vi "662xA Display Text.vi"(8 "error in (no error)":errorcluster, 9 "text message (TEST)":string="TEST", 10 "function (T:write)":bool=TRUE, 11 "VISA resource name":refnum<visa-resource-name>) -> (0 "error out":errorcluster, 3 "VISA resource name out":refnum<visa-resource-name>)   [LabVIEW 2020, in "Agilent 6XXX Series.lvlib"]
doc: "This function displays a text message on the front panel of the HP662XA series power supplies only."
uses:
  <instrlib>/Agilent 6XXX Series/Agilent 6XXX Series.lvlib
panel:
  # "HP662XA series only"
  # "write message\nclear message"
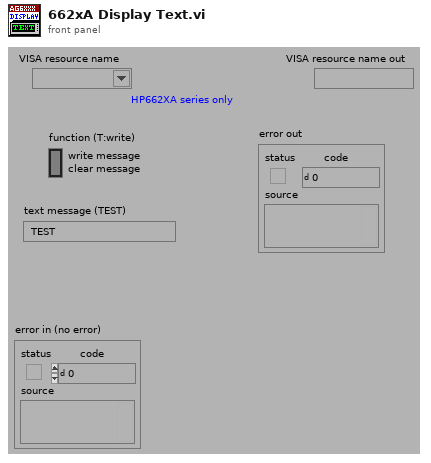
[diagram p1: front panel]
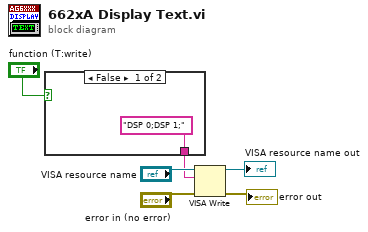
[diagram p0: block diagram]
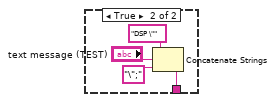
[diagram p2: hidden frame]
diagram:
  n1 = case shown="False" "function (T:write)" {
    tunnel: ["DSP 0;DSP 1;" w8] -> w1
    frame False {
    }
    frame True {
      n2 = Concatenate Strings("DSP \"", "text message (TEST)", "\";") -> (w8:string)
    }
  }
  n3 = VISA Write(VISA resource name="VISA resource name", write buffer=w1, error in (no error)="error in (no error)") -> (VISA resource name out=→"VISA resource name out":refnum<visa-resource-name>, error out=→"error out":errorcluster)  [unwired: 1 out]
